vi "FastBeamMode.vi"() -> ()   [LabVIEW 2021]
uses:
  C:/Users/Raymond_Su/Desktop/X410 Integration/FastBeamControl/FastBeamControl/BBoxAPI.dll
  kernel32.dll
panel:
  out "current state":i32
  out "SN":string
  out "Init":i32(ring) items=["OK"=0, "WARNING"=1, "ERROR"=2, "NO_RESPONSE"=3, "ERROR_GET_SN"=10, "ERROR_DEV_TYPE"=11, "ERROR_INIT_OBJECT"=12, "ERROR_DEV_NOT_INIT"=13, "ERROR_METHOD_NOT_FOUND"=14, "ERROR_REFLECTION"=15, "ERROR_POWER"=16, "ERROR_SCAN_NOT_FOUND"=17, "ERROR_UNMATCH_RETURN_TYPE"=18, "ERROR_NETWORK_NOT_INIT"=20, "ERROR_NETWORK_INIT"=21, "ERROR_NETWORK_CONNECT_TIMEOUT"=22, "ERROR_DISCONNECT"=23, "ERROR_SOCKET"=24, "ERROR_SEND_CMD"=25, "ERROR_RESP_CMD"=26, "ERROR_DEV_COUNT_ZERO"=30, "ERROR_DEV_DUMMY_FUNC"=31, "ERROR_CMD"=40, "ERROR_CMD_INIT"=41, "ERROR_BF_AAKIT"=100, "ERROR_BF_NO_AAKIT"=101, "ERROR_BF_CALI_PATH"=102, "ERROR_BF_BEAMXY"=103, "ERROR_BF_GEN"=104, "ERROR_BF_TRMODE"=105, "STATUS_BF_LOAD_CALI_INCOMPLTE"=106, "ERROR_BF_LOAD_CALI_PARSE_FAILED"=107, "ERROR_BF_UNLOAD_CALI"=108, "ERROR_BF_CALI_VERSION_UNSUPPORTED"=109, "ERROR_BF_CALI_DATA_NOT_FOUND"=110, "ERROR_FREQ_EQUATION"=250, "ERROR_PLO_CRC"=251, "WARNING_HARMONIC"=252, "ERROR_HARMONIC_BLOCK"=253, "ERROR_FW_UPGRADE_IP_INVALID"=300, "ERROR_FW_VERSION_NOT_SUPPORT"=301]
  out "getFrequencyList":string[](array[string])
  out "checkCaliTableLocation":bool
  out "Console Log":string
  out "status":bool
  out "Target SN":string
  in  "Device SN":string="B00000000-00"
  out "SN_is_match":bool
  out "ScanResult":string[](array[string])
  out "Target AAKit Name":string
  out "selectAAKit":i32(ring)=13 items=["OK"=0, "WARNING"=1, "ERROR"=2, "NO_RESPONSE"=3, "ERROR_GET_SN"=10, "ERROR_DEV_TYPE"=11, "ERROR_INIT_OBJECT"=12, "ERROR_DEV_NOT_INIT"=13, "ERROR_METHOD_NOT_FOUND"=14, "ERROR_REFLECTION"=15, "ERROR_POWER"=16, "ERROR_NETWORK_NOT_INIT"=20, "ERROR_NETWORK_INIT"=21, "ERROR_NETWORK_CONNECT_TIMEOUT"=22, "ERROR_DISCONNECT"=23, "ERROR_SOCKET"=24, "ERROR_SEND_CMD"=25, "ERROR_RESP_CMD"=26, "ERROR_DEV_COUNT_ZERO"=30, "ERROR_CMD"=40, "ERROR_CMD_INIT"=41, "ERROR_BF_AAKIT"=100, "ERROR_BF_NO_AAKIT"=101, "ERROR_BF_CALI_PATH"=102, "ERROR_BF_BEAMXY"=103, "ERROR_BF_GEN"=104, "ERROR_BF_TRMODE"=105, "STATUS_BF_LOAD_CALI_INCOMPLTE"=106, "ERROR_BF_LOAD_CALI_PARSE_FAILED"=107, "ERROR_FREQ_EQUATION"=250, "ERROR_PLO_CRC"=251, "WARNING_HARMONIC"=252, "ERROR_HARMONIC_BLOCK"=253]
  in  "Fast BeamMode Enable":bool=TRUE
  out "getAAKitList":string[](array[string])
  in  "Target AAKit Index":i32 min=1 max=2 step=1
  in  "Target Freq Index":i32 min=1 max=2 step=1
  out "setOperatingFreq":i32(ring)=13 items=["OK"=0, "WARNING"=1, "ERROR"=2, "NO_RESPONSE"=3, "ERROR_GET_SN"=10, "ERROR_DEV_TYPE"=11, "ERROR_INIT_OBJECT"=12, "ERROR_DEV_NOT_INIT"=13, "ERROR_METHOD_NOT_FOUND"=14, "ERROR_REFLECTION"=15, "ERROR_POWER"=16, "ERROR_NETWORK_NOT_INIT"=20, "ERROR_NETWORK_INIT"=21, "ERROR_NETWORK_CONNECT_TIMEOUT"=22, "ERROR_DISCONNECT"=23, "ERROR_SOCKET"=24, "ERROR_SEND_CMD"=25, "ERROR_RESP_CMD"=26, "ERROR_DEV_COUNT_ZERO"=30, "ERROR_CMD"=40, "ERROR_CMD_INIT"=41, "ERROR_BF_AAKIT"=100, "ERROR_BF_NO_AAKIT"=101, "ERROR_BF_CALI_PATH"=102, "ERROR_BF_BEAMXY"=103, "ERROR_BF_GEN"=104, "ERROR_BF_TRMODE"=105, "STATUS_BF_LOAD_CALI_INCOMPLTE"=106, "ERROR_BF_LOAD_CALI_PARSE_FAILED"=107, "ERROR_FREQ_EQUATION"=250, "ERROR_PLO_CRC"=251, "WARNING_HARMONIC"=252, "ERROR_HARMONIC_BLOCK"=253]
  out "Set_Fast_Parallel_Mode":i32(ring) items=["OK"=0, "WARNING"=1, "ERROR"=2, "NO_RESPONSE"=3, "ERROR_GET_SN"=10, "ERROR_DEV_TYPE"=11, "ERROR_INIT_OBJECT"=12, "ERROR_DEV_NOT_INIT"=13, "ERROR_METHOD_NOT_FOUND"=14, "ERROR_REFLECTION"=15, "ERROR_POWER"=16, "ERROR_SCAN_NOT_FOUND"=17, "ERROR_UNMATCH_RETURN_TYPE"=18, "ERROR_NETWORK_NOT_INIT"=20, "ERROR_NETWORK_INIT"=21, "ERROR_NETWORK_CONNECT_TIMEOUT"=22, "ERROR_DISCONNECT"=23, "ERROR_SOCKET"=24, "ERROR_SEND_CMD"=25, "ERROR_RESP_CMD"=26, "ERROR_DEV_COUNT_ZERO"=30, "ERROR_DEV_DUMMY_FUNC"=31, "ERROR_CMD"=40, "ERROR_CMD_INIT"=41, "ERROR_BF_AAKIT"=100, "ERROR_BF_NO_AAKIT"=101, "ERROR_BF_CALI_PATH"=102, "ERROR_BF_BEAMXY"=103, "ERROR_BF_GEN"=104, "ERROR_BF_TRMODE"=105, "STATUS_BF_LOAD_CALI_INCOMPLTE"=106, "ERROR_BF_LOAD_CALI_PARSE_FAILED"=107, "ERROR_BF_UNLOAD_CALI"=108, "ERROR_BF_CALI_VERSION_UNSUPPORTED"=109, "ERROR_BF_CALI_DATA_NOT_FOUND"=110, "ERROR_FREQ_EQUATION"=250, "ERROR_PLO_CRC"=251, "WARNING_HARMONIC"=252, "ERROR_HARMONIC_BLOCK"=253, "ERROR_FW_UPGRADE_IP_INVALID"=300, "ERROR_FW_VERSION_NOT_SUPPORT"=301]
  in  "Start":bool=TRUE
  in  "Set Current Working Directory":path
  out "Get Current Working Directory":path
  out "Exists Table Filenames":string[](array[string])
  # "Notice:\n\nThe Set / Get Current Working Diectory Path must be the sample code directory path : bbox-api\\example\\BBoxOne Series\\LabVIEW\\\n\nMust exist\n\n1. bbox-api\\example\\BBoxOne Series\\LabVIEW\\BBoxAPI.dll\n\n2. bbox-api\\example\\BBoxOne Series\\LabVIEW\\files\\\n\n3. bbox-api\\example\\BBoxOne Series\\LabVIEW\\logs\\"
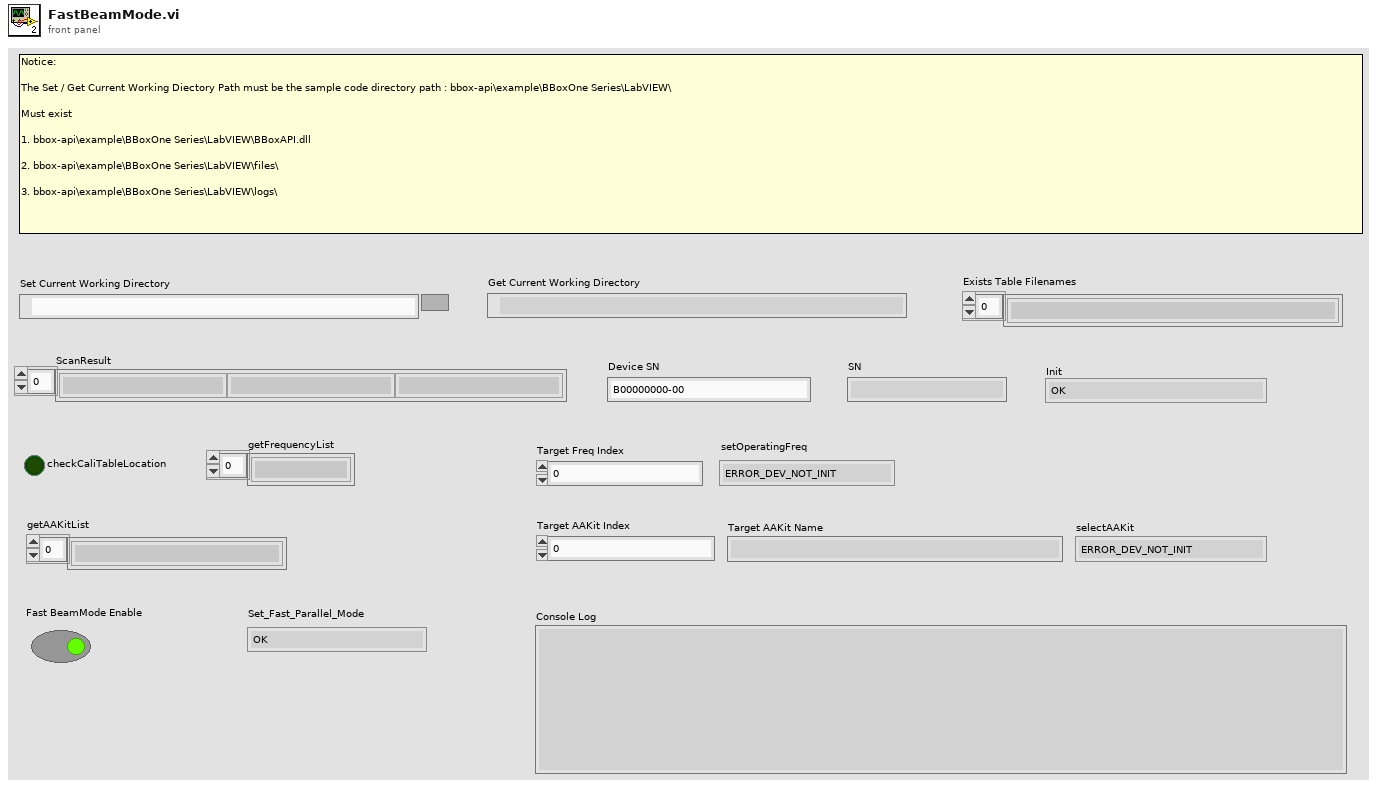
[diagram p1: front panel]
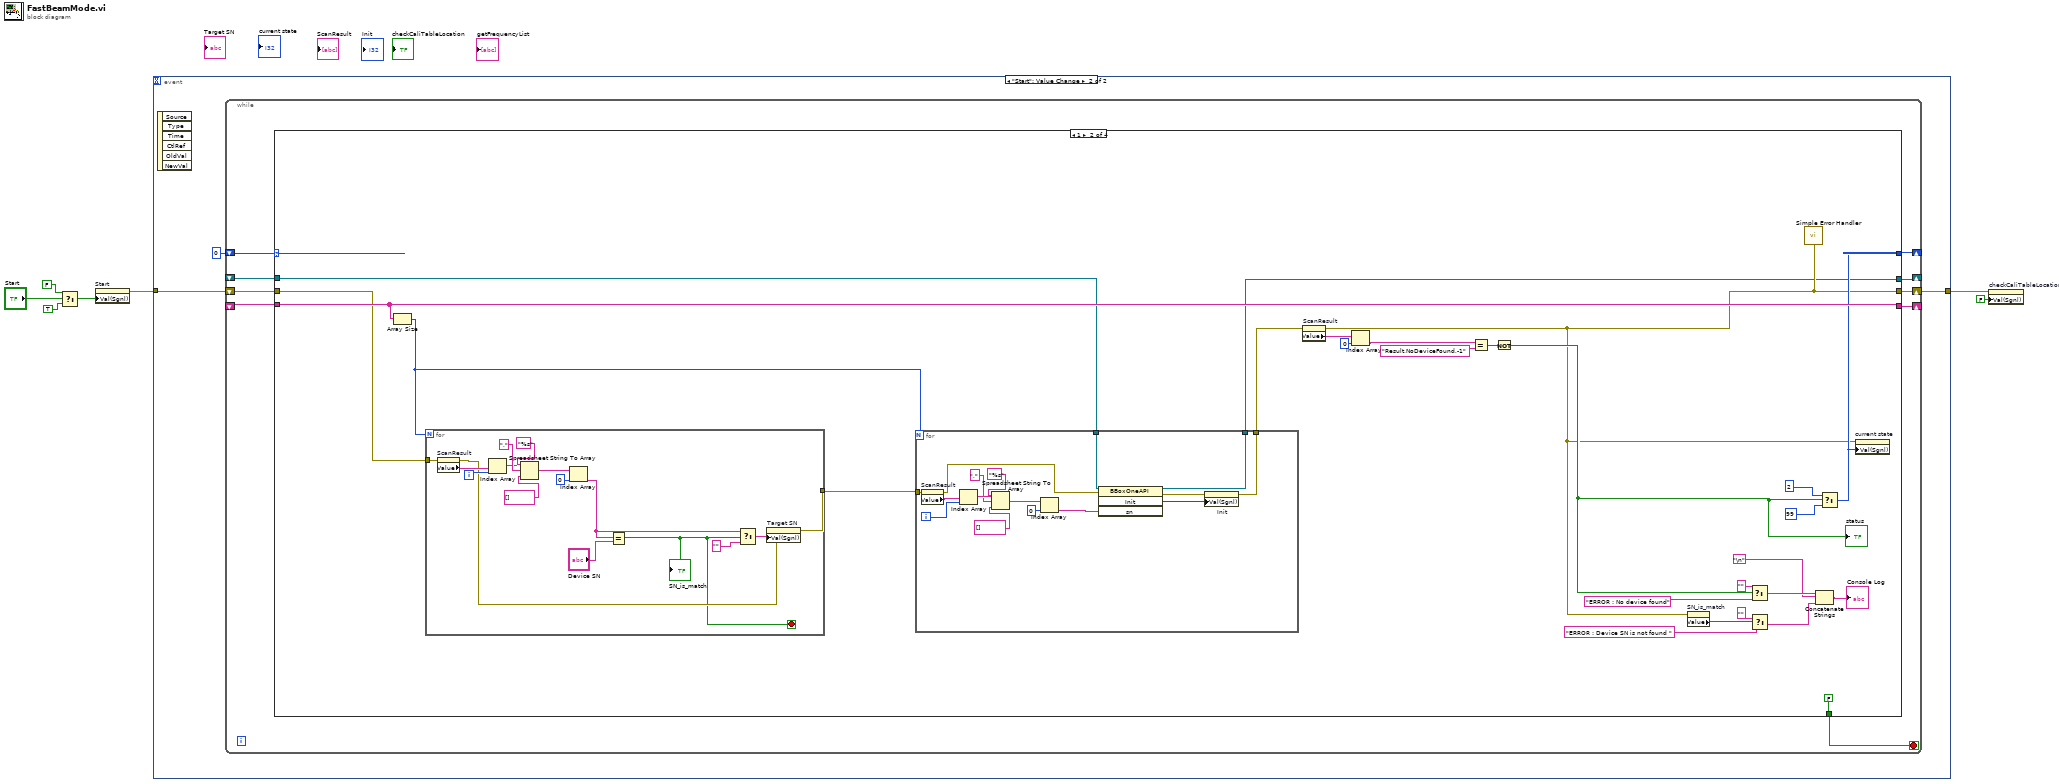
[diagram p0: block diagram]
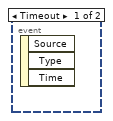
[diagram p2: hidden frame]
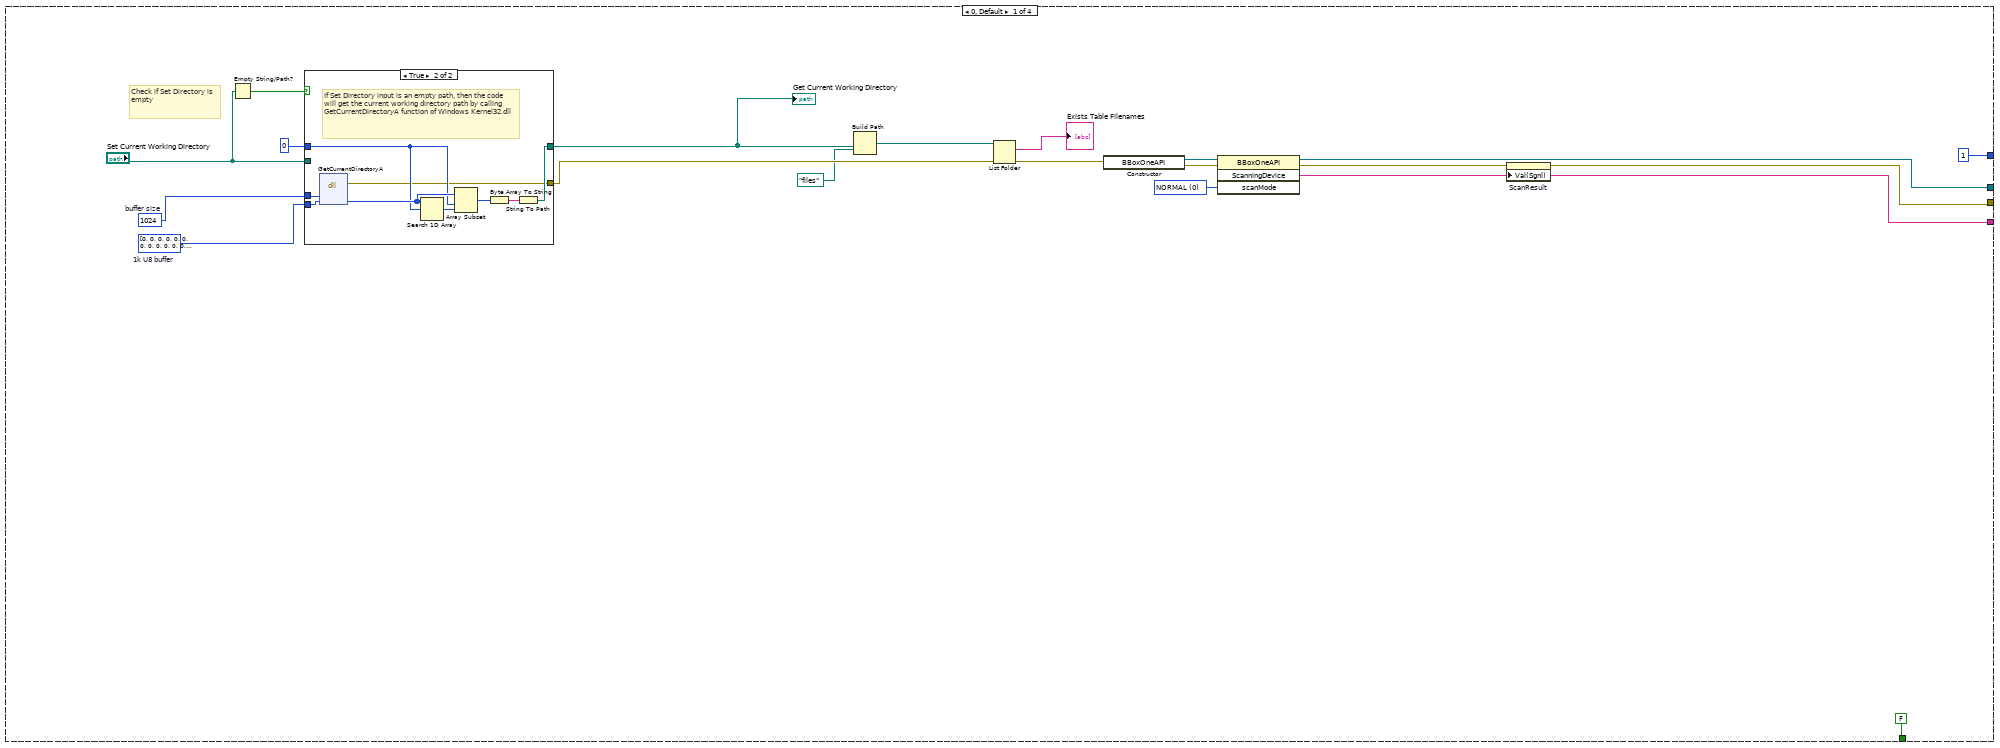
[diagram p3: hidden frame]
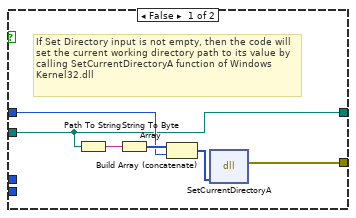
[diagram p4: hidden frame]
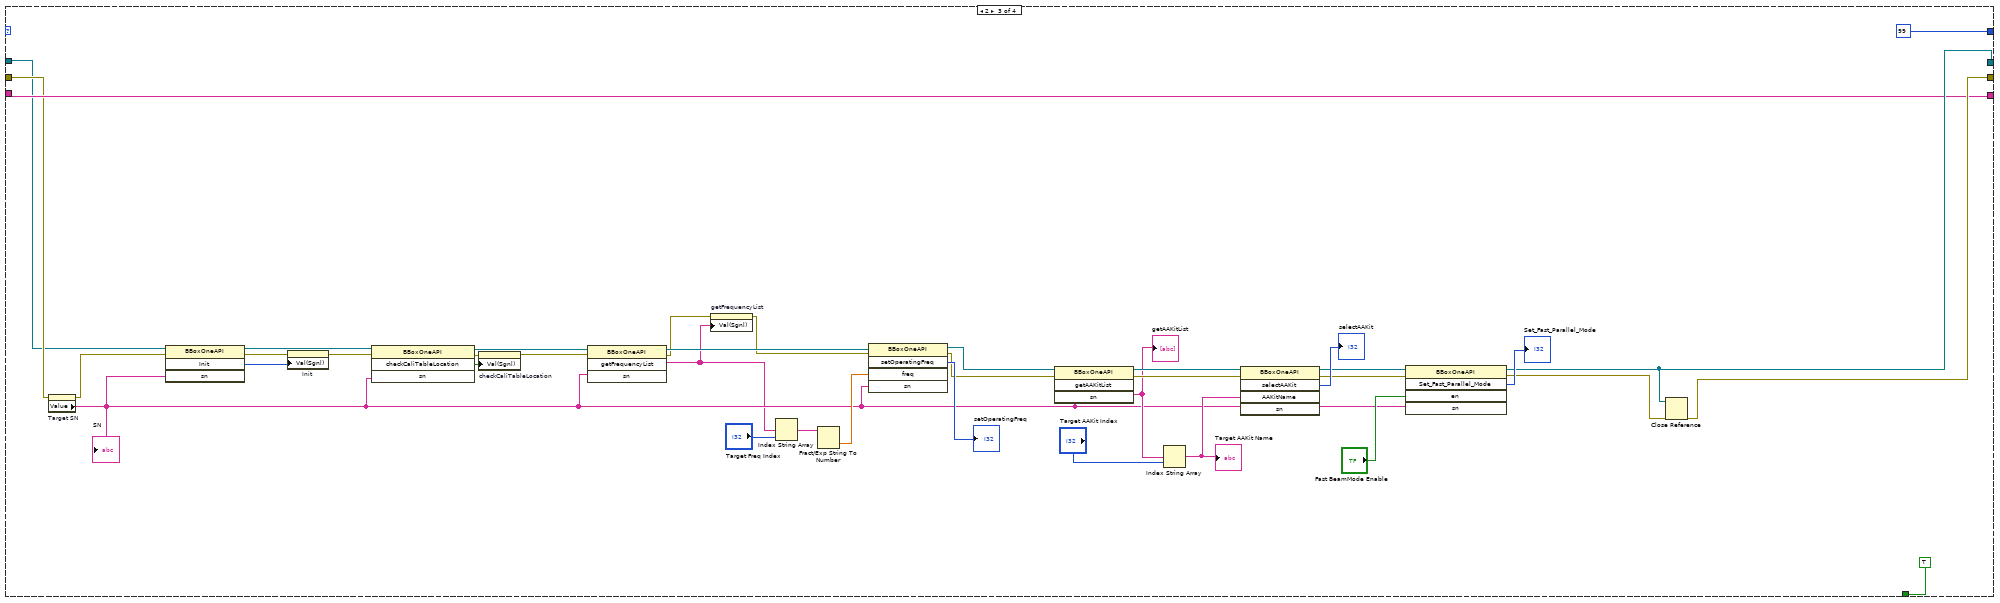
[diagram p5: hidden frame]
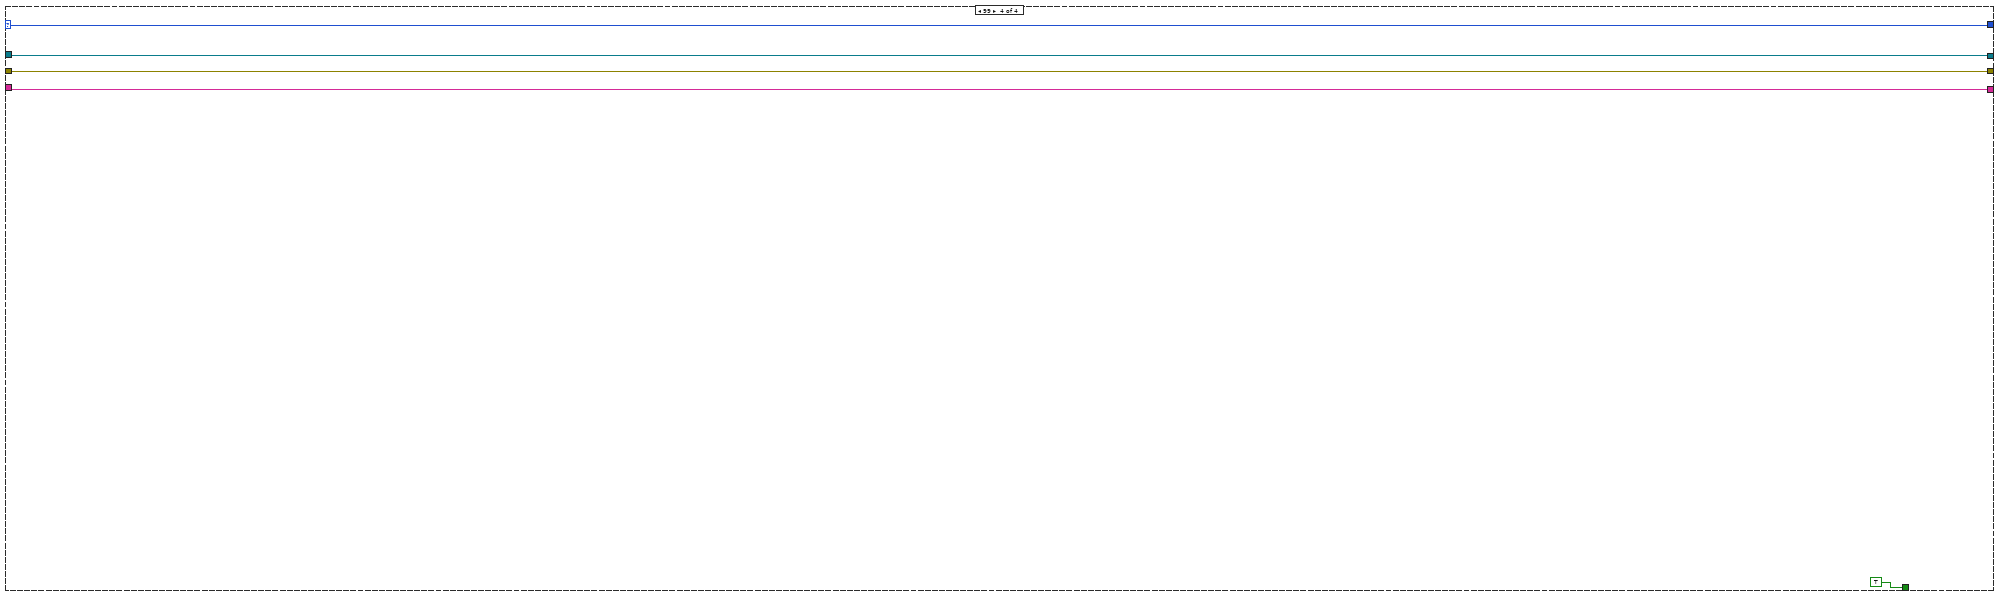
[diagram p6: hidden frame]
diagram:
  n1 = Select(t=FALSE ("Value (Signaling)"), s="Start", f=TRUE) -> (s? t:f=w4:bool)
  n2 = property on="Start" class="Bool (strict)"("Val(Sgnl)"=w4) -> (error out=w3:errorcluster)  [unwired: 2 in, 1 out]
  n3 = event shown="[1] \"Start\": Value Change" {
    selector: _ -> [_ _]
    dyn-events: _ -> [_ _]
    timeout: _ -> [_ _]
    tunnel: w3 -> [_ w10]
    tunnel: [_ w8] -> w2
    event Timeout {
      n4 = event-data() -> ()  [unwired: 1 in, 3 out]
    }
    event "Start": Value Change {
      n5 = event-data() -> ()  [unwired: 1 in, 6 out]
      n6 = while {
        shift-right: [w18] -> _
        shift-left: 0 -> [w19]
        shift-right: [w16] -> w8
        shift-left: w10 -> [w13]
        shift-right: [w15] -> _
        shift-left: _ -> [w14]
        shift-right: [w11] -> _
        shift-left: _ -> [w12]
        stop <- w17 stop-if-true
        n7 = case shown="1" w19 {
          selector: w19 -> [_ _ _ w155]
          tunnel: [1 w63 99 w155] -> w18
          tunnel: [FALSE FALSE TRUE TRUE] -> w17
          tunnel: [w20 w58 w132 w152] -> w16
          tunnel: [w21 w56 w131 w153] -> w15
          tunnel: w14 -> [_ w57 w124 w153]
          tunnel: w13 -> [_ w67 w128 w152]
          tunnel: w12 -> [_ w68 w129 w151]
          tunnel: [w23 w68 w129 w151] -> w11
          frame 0, Default {
            w31 = 1024  # buffer size
            w30 = u8[] [0, 0, 0, 0, 0, 0, 0, 0, 0, 0, 0, 0, 0, 0, 0, 0, 0, 0, 0, 0, 0, 0, 0, 0, 0, 0, 0, 0, 0, 0, 0, 0, 0, 0, 0, 0, 0, 0, 0, 0, 0, 0, 0, 0, 0, 0, 0, 0, 0, 0, 0, 0, 0, 0, 0, 0, 0, 0, 0, 0, 0, 0, 0, 0, 0, 0, 0, 0, 0, 0, 0, 0, 0, 0, 0, 0, 0, 0, 0, 0, 0, 0, 0, 0, 0, 0, 0, 0, 0, 0, 0, 0, 0, 0, 0, 0, 0, 0, 0, 0, 0, 0, 0, 0, 0, 0, 0, 0, 0, 0, 0, 0, 0, 0, 0, 0, 0, 0, 0, 0, 0, 0, 0, 0, 0, 0, 0, 0, 0, 0, 0, 0, 0, 0, 0, 0, 0, 0, 0, 0, 0, 0, 0, 0, 0, 0, 0, 0, 0, 0, 0, 0, 0, 0, 0, 0, 0, 0, 0, 0, 0, 0, 0, 0, 0, 0, 0, 0, 0, 0, 0, 0, 0, 0, 0, 0, 0, 0, 0, 0, 0, 0, 0, 0, 0, 0, 0, 0, 0, 0, 0, 0, 0, 0, 0, 0, 0, 0, 0, 0, 0, 0, 0, 0, 0, 0, 0, 0, 0, 0, 0, 0, 0, 0, 0, 0, 0, 0, 0, 0, 0, 0, 0, 0, 0, 0, 0, 0, 0, 0, 0, 0, 0, 0, 0, 0, 0, 0, 0, 0, 0, 0, 0, 0, 0, 0, 0, 0, 0, 0, 0, 0, 0, 0, 0, 0, 0, 0, 0, 0, 0, 0, 0, 0, 0, 0, 0, 0, 0, 0, 0, 0, 0, 0, 0, 0, 0, 0, 0, 0, 0, 0, 0, 0, 0, 0, 0, 0, 0, 0, 0, 0, 0, 0, 0, 0, 0, 0, 0, 0, 0, 0, 0, 0, 0, 0, 0, 0, 0, 0, 0, 0, 0, 0, 0, 0, 0, 0, 0, 0, 0, 0, 0, 0, 0, 0, 0, 0, 0, 0, 0, 0, 0, 0, 0, 0, 0, 0, 0, 0, 0, 0, 0, 0, 0, 0, 0, 0, 0, 0, 0, 0, 0, 0, 0, 0, 0, 0, 0, 0, 0, 0, 0, 0, 0, 0, 0, 0, 0, 0, 0, 0, 0, 0, 0, 0, 0, 0, 0, 0, 0, 0, 0, 0, 0, 0, 0, 0, 0, 0, 0, 0, 0, 0, 0, 0, 0, 0, 0, 0, 0, 0, 0, 0, 0, 0, 0, 0, 0, 0, 0, 0, 0, 0, 0, 0, 0, 0, 0, 0, 0, 0, 0, 0, 0, 0, 0, 0, 0, 0, 0, 0, 0, 0, 0, 0, 0, 0, 0, 0, 0, 0, 0, 0, 0, 0, 0, 0, 0, 0, 0, 0, 0, 0, 0, 0, 0, 0, 0, 0, 0, 0, 0, 0, 0, 0, 0, 0, 0, 0, 0, 0, 0, 0, 0, 0, 0, 0, 0, 0, 0, 0, 0, 0, 0, 0, 0, 0, 0, 0, 0, 0, 0, 0, 0, 0, 0, 0, 0, 0, 0, 0, 0, 0, 0, 0, 0, 0, 0, 0, 0, 0, 0, 0, 0, 0, 0, 0, 0, 0, 0, 0, 0, 0, 0, 0, 0, 0, 0, 0, 0, 0, 0, 0, 0, 0, 0, 0, 0, 0, 0, 0, 0, 0, 0, 0, 0, 0, 0, 0, 0, 0, 0, 0, 0, 0, 0, 0, 0, 0, 0, 0, 0, 0, 0, 0, 0, 0, 0, 0, 0, 0, 0, 0, 0, 0, 0, 0, 0, 0, 0, 0, 0, 0, 0, 0, 0, 0, 0, 0, 0, 0, 0, 0, 0, 0, 0, 0, 0, 0, 0, 0, 0, 0, 0, 0, 0, 0, 0, 0, 0, 0, 0, 0, 0, 0, 0, 0, 0, 0, 0, 0, 0, 0, 0, 0, 0, 0, 0, 0, 0, 0, 0, 0, 0, 0, 0, 0, 0, 0, 0, 0, 0, 0, 0, 0, 0, 0, 0, 0, 0, 0, 0, 0, 0, 0, 0, 0, 0, 0, 0, 0, 0, 0, 0, 0, 0, 0, 0, 0, 0, 0, 0, 0, 0, 0, 0, 0, 0, 0, 0, 0, 0, 0, 0, 0, 0, 0, 0, 0, 0, 0, 0, 0, 0, 0, 0, 0, 0, 0, 0, 0, 0, 0, 0, 0, 0, 0, 0, 0, 0, 0, 0, 0, 0, 0, 0, 0, 0, 0, 0, 0, 0, 0, 0, 0, 0, 0, 0, 0, 0, 0, 0, 0, 0, 0, 0, 0, 0, 0, 0, 0, 0, 0, 0, 0, 0, 0, 0, 0, 0, 0, 0, 0, 0, 0, 0, 0, 0, 0, 0, 0, 0, 0, 0, 0, 0, 0, 0, 0, 0, 0, 0, 0, 0, 0, 0, 0, 0, 0, 0, 0, 0, 0, 0, 0, 0, 0, 0, 0, 0, 0, 0, 0, 0, 0, 0, 0, 0, 0, 0, 0, 0, 0, 0, 0, 0, 0, 0, 0, 0, 0, 0, 0, 0, 0, 0, 0, 0, 0, 0, 0, 0, 0, 0, 0, 0, 0, 0, 0, 0, 0, 0, 0, 0, 0, 0, 0, 0, 0, 0, 0, 0, 0, 0, 0, 0, 0, 0, 0, 0, 0, 0, 0, 0, 0, 0, 0, 0, 0, 0, 0, 0, 0, 0, 0, 0, 0, 0, 0, 0, 0, 0, 0, 0, 0, 0, 0, 0, 0, 0, 0, 0, 0, 0, 0, 0, 0, 0, 0, 0, 0, 0, 0, 0, 0, 0, 0, 0, 0, 0, 0, 0, 0, 0, 0, 0, 0, 0, 0, 0, 0, 0, 0, 0, 0, 0, 0, 0, 0, 0, 0, 0, 0, 0, 0, 0, 0, 0, 0, 0, 0, 0, 0, 0, 0, 0, 0, 0, 0, 0, 0, 0, 0, 0, 0, 0, 0, 0, 0, 0, 0, 0, 0, 0, 0, 0, 0, 0, 0, 0, 0, 0, 0, 0, 0, 0, 0, 0, 0, 0, 0, 0, 0, 0, 0, 0, 0, 0, 0, 0, 0, 0, 0, 0, 0, 0, 0, 0, 0, 0, 0, 0, 0, 0, 0, 0, 0, 0, 0, 0, 0, 0, 0, 0, 0, 0, 0, 0, 0, 0, 0, 0, 0, 0, 0, 0, 0, 0, 0, 0, 0, 0, 0]  # 1k U8 buffer
            w29 = 0 items=["NORMAL", "FAST"] ("scanMode")
            # "Check if Set Directory is empty"
            n8 = Empty String/Path?(string/path="Set Current Working Directory") -> (empty?=w36:bool)
            n9 = case shown="True" w36 {
              tunnel: "Set Current Working Directory" -> [w41 _]
              tunnel: u8 0 -> [w43 w50]
              tunnel: w31 -> [_ w49]
              tunnel: w30 -> [_ w48]
              tunnel: [w41 w47] -> w25
              tunnel: [w40 w46] -> w38
              frame False {
                # "If Set Directory input is not empty, then the code will set the current working directory path to its value by calling SetCurrentDirectoryA function of Windows Kernel32.dll"
                n10 = Path To String(path=w41) -> (string=w42:string)
                n11 = String To Byte Array(string=w42) -> (unsigned byte array=w45:u8[])
                n12 = Build Array (concatenate)(w45, w43) -> (w44:u8[])
                n13 = dll-call lib="Kernel32.dll" fn="SetCurrentDirectoryA" label="Kernel32.dll - \nSetCurrentDirectoryA"("lpPathName"=w44) -> (error out=w40:errorcluster)  [unwired: 4 in, 2 out]
              }
              frame True {
                # "If Set Directory input is an empty path, then the code will get the current working directory path by calling GetCurrentDirectoryA function of Windows Kernel32.dll"
                n14 = dll-call lib="kernel32.dll" fn="GetCurrentDirectoryA" label="Kernel32.dll - \nGetCurrentDirectoryA"("nBufferLength"=w49, "lpBuffer"=w48) -> (error out=w46:errorcluster, "lpBuffer"=w53:u8[])  [unwired: 4 in, 2 out]
                n15 = Search 1D Array(1D array=w53, element=w50) -> (index of element=w54:i32)  [unwired: 1 out]
                n16 = Array Subset(array=w53, index=w50, length=w54) -> (w51:u8[])
                n17 = Byte Array To String(unsigned byte array=w51) -> (string=w52:string)
                n18 = String To Path(string=w52) -> (path=w47:path)
              }
            }
            "Get Current Working Directory" <- w25
            n19 = Build Path(base path=w25, name or relative path=path "files") -> (appended path=w37:path)
            n20 = List Folder(path=w37, error in=w38) -> (filenames=→"Exists Table Filenames":string[], error out=w39:errorcluster)  [unwired: 2 in, 2 out]
            n21 = constructor class="BBoxOneAPI"(error in=w39) -> (reference out=w34:refnum<k24>, error out=w35:errorcluster)  [unwired: 2 in, 1 out]
            n22 = invoke class="BBoxOneAPI" method="ScanningDevice"(reference=w34, error in=w35, "scanMode"=w29) -> (reference out=w21:refnum<k24>, error out=w22:errorcluster, "ScanningDevice"=w23:string[])  [unwired: 1 in, 1 out]
            n23 = property on="ScanResult" class="Arr (strict)"(error in=w22, "Val(Sgnl)"=w23) -> (error out=w20:errorcluster)  [unwired: 1 in, 1 out]
          }
          frame 1 {
            n24 = Array Size(array=w68) -> (size(s)=w55:i32)
            n25 = for {
              N: w55 -> [_]
              tunnel: w67 -> [w102]
              tunnel: [w99] -> w59
              i -> [w107]
              stop <- w97 stop-if-true
              n26 = property on="ScanResult" class="Arr (strict)"(error in=w102) -> (error out=w100:errorcluster, "Value"=w103:string[])  [unwired: 1 in, 1 out]
              n27 = Index Array(array=w103, index=w107) -> (element=w110:string)
              n28 = Spreadsheet String To Array(delimiter (Tab)=",", format string="%s", spreadsheet string=w110, array type (2D Dbl)=string[] []) -> (array=w106:string[])
              n29 = Index Array(array=w106, index=0) -> (element=w98:string)
              n30 = Equal?(x=w98, y="Device SN") -> (x = y?=w97:bool)
              "SN_is_match" <- w97
              n31 = Select(t=w98, s=w97, f="") -> (s? t:f=w101:string)
              n32 = property on="Target SN" class="Str"(error in=w100, "Val(Sgnl)"=w101) -> (error out=w99:errorcluster)  [unwired: 1 in, 1 out]
            }
            n33 = for {
              N: w55 -> [_]
              tunnel: w59 -> [w87]
              tunnel: [w82] -> w58
              tunnel: w57 -> [w85]
              tunnel: [w84] -> w56
              i -> [w91]
              n34 = property on="ScanResult" class="Arr (strict)"(error in=w87) -> (error out=w86:errorcluster, "Value"=w92:string[])  [unwired: 1 in, 1 out]
              n35 = Index Array(array=w92, index=w91) -> (element=w96:string)
              n36 = Spreadsheet String To Array(delimiter (Tab)=",", format string="%s", spreadsheet string=w96, array type (2D Dbl)=string[] []) -> (array=w93:string[])
              n37 = Index Array(array=w93, index=0) -> (element=w88:string)
              n38 = invoke class="BBoxOneAPI" method="Init"(reference=w85, error in=w86, "sn"=w88) -> (reference out=w84:refnum<k24>, error out=w83:errorcluster, "Init"=w81:i32)  [unwired: 1 in, 1 out]
              n39 = property on="Init" class="Ring (strict)"(error in=w83, "Val(Sgnl)"=w81) -> (error out=w82:errorcluster)  [unwired: 1 in, 1 out]
            }
            n40 = property on="ScanResult" class="Arr (strict)"(error in=w58) -> ("Value"=w66:string[])  [unwired: 1 in, 2 out]
            n41 = Index Array(array=w66, index=0) -> (element=w65:string)
            n42 = Equal?(x=w65, y="Result,NoDeviceFound,-1") -> (x = y?=w78:bool)
            n43 = Not(x=w78) -> (.not. x?=w60:bool)
            "status" <- w60
            n44 = property on="SN_is_match" class="Bool (strict)"(error in=w58) -> ("Value"=w69:bool)  [unwired: 1 in, 2 out]
            n45 = Select(t="" ("y"), s=w60, f="ERROR : No device found" ("y")) -> (s? t:f=w73:string)
            n46 = Select(t="" ("y"), s=w69, f="ERROR : Device SN is not found " ("y")) -> (s? t:f=w61:string)
            n47 = call <vilib>:"Simple Error Handler.vi"("error in (no error)"=w58) -> ()  [unwired: 4 in, 5 out]
            n48 = Concatenate Strings(w73, "\n", w61) -> (→"Console Log":string)
            n49 = Select(t=2, s=w60, f=99) -> (s? t:f=w63:i32)
            n50 = property on="current state" class="DigNum (strict)"(error in=w58, "Val(Sgnl)"=w63) -> ()  [unwired: 1 in, 2 out]
          }
          frame 2 {
            n51 = property on="Target SN" class="Str"(error in=w128) -> (error out=w123:errorcluster, "Value"=w122:string)  [unwired: 1 in, 1 out]
            "SN" <- w122
            n52 = invoke class="BBoxOneAPI" method="Init"(reference=w124, error in=w123, "sn"=w122) -> (reference out=w127:refnum<k24>, error out=w121:errorcluster, "Init"=w119:i32)  [unwired: 1 in, 1 out]
            n53 = property on="Init" class="Ring (strict)"(error in=w121, "Val(Sgnl)"=w119) -> (error out=w120:errorcluster)  [unwired: 1 in, 1 out]
            n54 = invoke class="BBoxOneAPI" method="checkCaliTableLocation"(reference=w127, error in=w120, "sn"=w122) -> (reference out=w126:refnum<k24>, error out=w118:errorcluster, "checkCaliTableLocation"=w116:bool)  [unwired: 1 in, 1 out]
            n55 = property on="checkCaliTableLocation" class="Bool (strict)"(error in=w118, "Val(Sgnl)"=w116) -> (error out=w117:errorcluster)  [unwired: 1 in, 1 out]
            n56 = invoke class="BBoxOneAPI" method="getFrequencyList"(reference=w126, error in=w117, "sn"=w122) -> (reference out=w125:refnum<k24>, error out=w115:errorcluster, "getFrequencyList"=w113:string[])  [unwired: 1 in, 1 out]
            n57 = property on="getFrequencyList" class="Arr (strict)"(error in=w115, "Val(Sgnl)"=w113) -> (error out=w114:errorcluster)  [unwired: 1 in, 1 out]
            n58 = Index String Array(1:"Target Freq Index", 2:w113) -> (0:w147:string)  [unwired: 1 in]
            n59 = Fract/Exp String To Number(string=w147) -> (number=w146:dbl)  [unwired: 3 in, 1 out]
            n60 = invoke class="BBoxOneAPI" method="setOperatingFreq"(reference=w125, error in=w114, "freq"=w146, "sn"=w122) -> (reference out=w135:refnum<k24>, error out=w134:errorcluster, "setOperatingFreq"=→"setOperatingFreq":i32)  [unwired: 1 in, 2 out]
            n61 = invoke class="BBoxOneAPI" method="getAAKitList"(reference=w135, error in=w134, "sn"=w122) -> (reference out=w139:refnum<k24>, error out=w138:errorcluster, "getAAKitList"=w137:string[])  [unwired: 1 in, 1 out]
            "getAAKitList" <- w137
            n62 = Index String Array(1:"Target AAKit Index", 2:w137) -> (0:w130:string)  [unwired: 1 in]
            "Target AAKit Name" <- w130
            n63 = invoke class="BBoxOneAPI" method="selectAAKit"(reference=w139, error in=w138, "AAKitName"=w130, "sn"=w122) -> (reference out=w141:refnum<k24>, error out=w140:errorcluster, "selectAAKit"=→"selectAAKit":i32)  [unwired: 1 in, 2 out]
            n64 = invoke class="BBoxOneAPI" method="Set_Fast_Parallel_Mode"(reference=w141, error in=w140, "en"="Fast BeamMode Enable", "sn"=w122) -> (reference out=w131:refnum<k24>, error out=w133:errorcluster, "Set_Fast_Parallel_Mode"=→"Set_Fast_Parallel_Mode":i32)  [unwired: 1 in, 2 out]
            n65 = Close Reference(reference=w131, error in (no error)=w133) -> (error out=w132:errorcluster)
          }
          frame 99 {
          }
        }
      }
    }
  }
  n66 = property on="checkCaliTableLocation" class="Bool (strict)"(error in=w2, "Val(Sgnl)"=FALSE ("Value (Signaling)")) -> ()  [unwired: 1 in, 2 out]
